vi "shift.vi"(8 "error in (no error)":errorcluster, 9 "deltaY[pixel]":i32, 10 "deltaX_[pixel]":i32, 11 "GObject in":refnum<class "GObject.lvclass">) -> (0 "error out":errorcluster, 3 "GObject out":refnum<class "GObject.lvclass">)   [LabVIEW 2023, in "TLC_Scripto.lvlib" / "GObject.lvclass"]
uses:
  GObject.lvclass
  Read position.vi
  Write position.vi
  GObject.lvclass/GObject.ctl
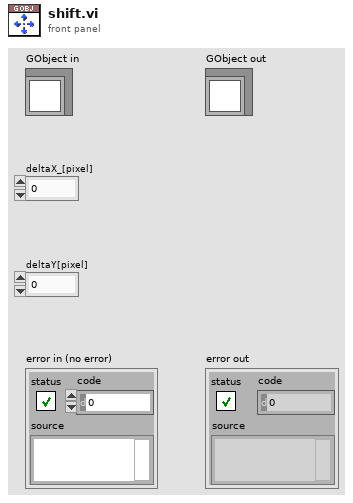
[diagram p1: front panel]
types:
  T1 = typedef "LVPositionTypeDef.ctl" = cluster{"Left":i32, "Top":i32}
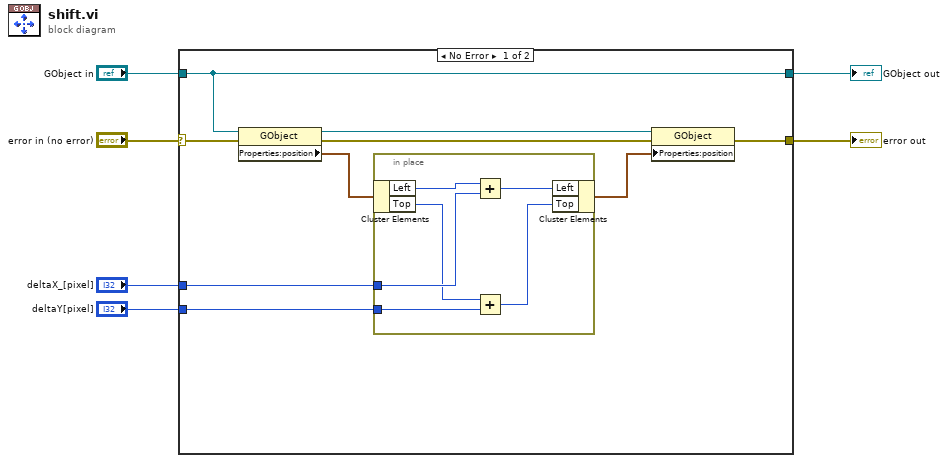
[diagram p0: block diagram]
diagram:
  n1 = case shown="No Error" "error in (no error)" {
    selector: "error in (no error)" -> [w13 w23]
    tunnel: [w12 w23] -> w5
    tunnel: [w7 w22] -> w3
    tunnel: "GObject in" -> [w7 w22]
    tunnel: "deltaX_[pixel]" -> [w9 _]
    tunnel: "deltaY[pixel]" -> [w8 _]
    frame No Error {
      n2 = property class="GObject"(reference=w7, error in=w13) -> (reference out=w15:refnum<class "GObject.lvclass">, error out=w14:errorcluster, "Properties:position"=w11:T1)
      n3 = in-place {
        in-place-border: w9 -> [w20]
        in-place-border: w8 -> [w16]
        n4 = in-place-cluster #1(w11) -> ("Left"=w21:i32, "Top"=w18:i32)
        n5 = Add(x=w21, y=w20) -> (x+y=w19:i32)
        n6 = Add(x=w18, y=w16) -> (x+y=w17:i32)
        n7 = in-place-cluster #1("Left"=w19, "Top"=w17) -> (w10:T1)
      }
      n8 = property class="GObject"(reference=w15, error in=w14, "Properties:position"=w10) -> (error out=w12:errorcluster)  [unwired: 1 out]
    }
    frame Error {
    }
  }
  "error out" <- w5
  "GObject out" <- w3
